vi "CreateArbWfrm.vi"(8 "error in (no error)":errorcluster, 11 "ClassIn":refnum<class "NiPxi6733.lvclass">) -> (0 "error out":errorcluster, 3 "ClassOut":refnum<class "NiPxi6733.lvclass">)   [LabVIEW 2014, in "FGenPlugins.lvlib" / "NiPxi6733.lvclass"]
uses:
  NiPxi6733.lvclass
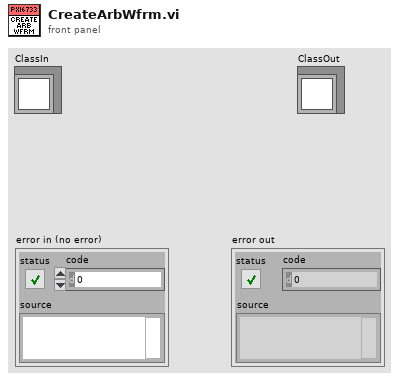
[diagram p1: front panel]
types:
  T1 = typedef "NISTFGenPlugins.lvlib/NISTFGenPluginsBase.lvclass/ArbWfrmParams.ctl" = cluster{"sWfrmHandle":string, "iSize":i32, "dData":dbl[], "dGain":dbl, "dOffset":dbl, "dSampleRate":dbl}
  T2 = typedef "FGenPlugins.lvlib/NISTFGenPluginsBase.lvclass/ChannelParamElement.ctl" = cluster{"sName":string, "eOperateMode":u16, "bEnabled":bool, "eOutputMode":u16, "iIndex":i32, "iNameBufferSize":i32, "fGain":dbl}
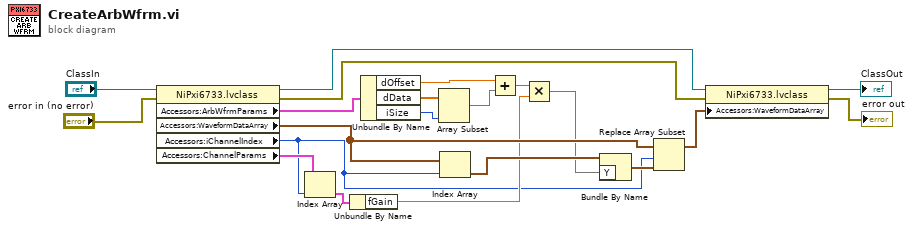
[diagram p0: block diagram]
diagram:
  n1 = property class="NiPxi6733.lvclass"(reference="ClassIn", error in="error in (no error)") -> (reference out=w10:refnum<class "NiPxi6733.lvclass">, error out=w12:errorcluster, "Accessors:ArbWfrmParams"=w18:T1, "Accessors:WaveformDataArray"=w11:waveform(dbl)[], "Accessors:iChannelIndex"=w1:i32, "Accessors:ChannelParams"=w8:T2[])
  n2 = Index Array(array=w8, index=w1) -> (element=w7:T2)
  n3 = Unbundle By Name(w7) -> ("fGain"=w3:dbl)
  n4 = Unbundle By Name(w18) -> ("dOffset"=w5:dbl, "dData"=w17:dbl[], "iSize"=w16:i32)
  n5 = Array Subset(array=w17, length=w16) -> (w6:dbl[])  [unwired: 1 in]
  n6 = Index Array(array=w11, index=w1) -> (element=w15:waveform(dbl))
  n7 = Add(x=w5, y=w6) -> (x+y=w4:dbl[])
  n8 = Multiply(x=w4, y=w3) -> (x*y=w2:dbl[])
  n9 = Bundle By Name(cluster=w15, "Y"=w2) -> (w14:waveform(dbl))
  n10 = Replace Array Subset(array=w11, new element=w14, index=w1) -> (w13:waveform(dbl)[])
  n11 = property class="NiPxi6733.lvclass"(reference=w10, error in=w12, "Accessors:WaveformDataArray"=w13) -> (reference out=→"ClassOut":refnum<class "NiPxi6733.lvclass">, error out=→"error out":errorcluster)
